vi "stampa_file.vi"(1 "Tensione":dbl[](array[numeric]), 2 "Tempo":dbl[](array[numeric]), 4 "Corrente":dbl[](array[numeric]), 6 "Corrente":dbl[](array[numeric]), 8 "error in (no error)":errorcluster, 9 "Tensione":dbl[](array[numeric]), 10 "Tempo":dbl[](array[numeric]), 11 "file path (dialog if empty)":path) -> (0 "error out":errorcluster, 3 "new file path (Not A Path if cancelled)":path)   [LabVIEW 2025]
uses:
  <vilib>/Utility/file.llb/Write Delimited Spreadsheet (string).vi
panel:
  in  "String 3":string="Corrente"
  in  "String 2":string="Tensione"
  in  "String":string="Tempo"
  out "F-format string":string[][](array[string])
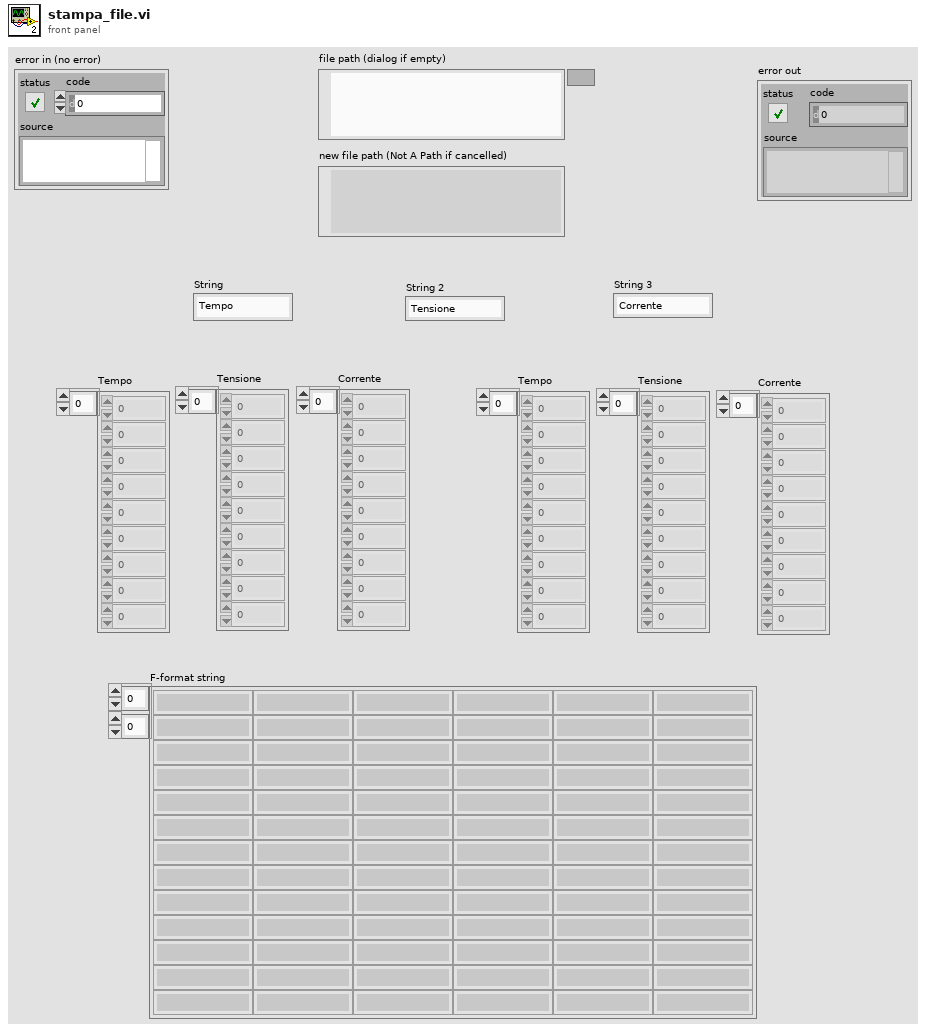
[diagram p1: front panel]
types:
  T1 = typedef "NI_Matrix.lvlib/RealMatrix.ctl" = dbl[][]
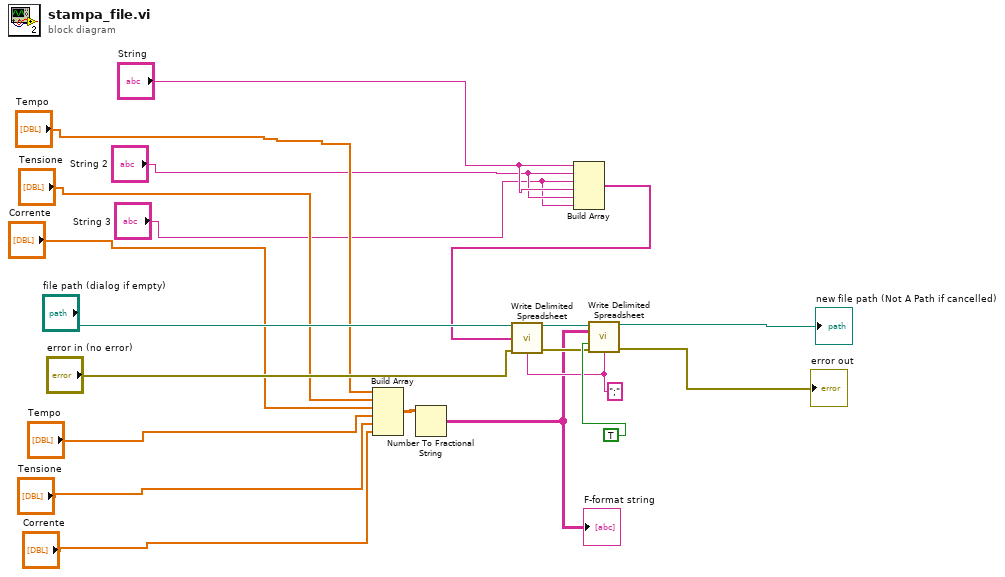
[diagram p0: block diagram]
diagram:
  w15 = ";" ("delimiter (\\t)")
  n1 = Build Array("Tempo", "Tensione", "Corrente", "Tempo", "Tensione", "Corrente") -> (w2:T1)
  n2 = Number To Fractional String(number=w2) -> (F-format string=w1:string[][])  [unwired: 3 in]
  "F-format string" <- w1
  n3 = Build Array("String", "String 2", "String 3", "String", "String 2", "String 3") -> (w13:string[])
  n4 = call-poly <vilib>:"Write Delimited Spreadsheet.vi"("file path (dialog if empty)"="file path (dialog if empty)", "1D data"=w13, "error in (no error)"="error in (no error)", "delimiter (\\t)"=w15) -> ("new file path (Not A Path if cancelled)"=w20:path, "error out"=w17:errorcluster)  [unwired: 10 in]
  n5 = call-poly <vilib>:"Write Delimited Spreadsheet.vi"("file path (dialog if empty)"=w20, "2D data"=w1, "append to file? (new file:F)"=TRUE, "error in (no error)"=w17, "delimiter (\\t)"=w15) -> ("new file path (Not A Path if cancelled)"=→"new file path (Not A Path if cancelled)":path, "error out"=→"error out":errorcluster)  [unwired: 9 in]
